vi "JSON Tags on Array.vi"(10 "Array Name":string, 11 "Element Name":string) -> (3 "Tag":T1)   [LabVIEW 2019, in "JSONtext.lvlib"]
uses:
  JSONtext.lvlib
  Tag Type.ctl
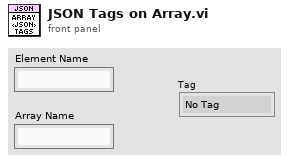
[diagram p1: front panel]
types:
  T1 = typedef "JSONtext.lvlib/Tag Type.ctl" = enum16{"No Tag", "<JSON>", "<JOBJ>"}
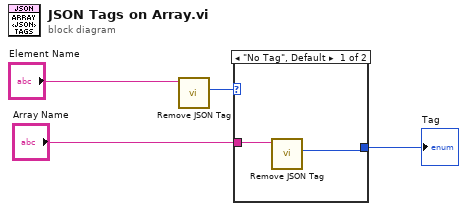
[diagram p0: block diagram]
diagram:
  n1 = call "Remove JSON Tag.vi"("Name"="Element Name") -> ("Tag"=w2:T1)  [unwired: 9 in, 1 out]
  n2 = case shown="\"No Tag\", Default" w2 {
    selector: w2 -> [_ w7]
    tunnel: "Array Name" -> [w6 _]
    tunnel: [w5 w7] -> w1
    frame "No Tag", Default {
      n3 = call "Remove JSON Tag.vi"("Name"=w6) -> ("Tag"=w5:T1)  [unwired: 9 in, 1 out]
    }
    frame "<JSON>" {
    }
  }
  "Tag" <- w1
